vi "Search for Array.vi"() -> ()   [LabVIEW 2020]
uses:
  <vilib>/Utility/file.llb/Read Delimited Spreadsheet (string).vi
panel:
  out "x+1":i32
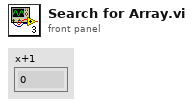
[diagram p1: front panel]
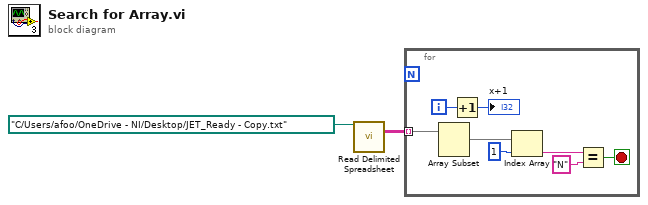
[diagram p0: block diagram]
diagram:
  n1 = call-poly <vilib>:"Read Delimited Spreadsheet.vi"("file path (dialog if empty)"=path "C:/Users/afoo/OneDrive - NI/Desktop/JET_Ready - Copy.txt") -> ("all rows"=w1:string[][])  [unwired: 9 in, 5 out]
  n2 = for {
    tunnel: w1 -> [w10] mode=indexing
    i -> [w4]
    stop <- w5 stop-if-true
    n3 = Array Subset(array=w10) -> (w9:string[])  [unwired: 2 in]
    n4 = Increment(x=w4) -> (x+1=→"x+1":i32)
    n5 = Index Array(array=w9, index=1) -> (element=w7:string)
    n6 = Equal?(x=w7, y="N" ("regular expression")) -> (x = y?=w5:bool)
  }
